vi "Initialize Instrument.vi"(8 "error in (no error)":errorcluster, 10 "Reset":bool, 11 "RS Z2X in":refnum<class "RS Z2X.lvclass">) -> (0 "error out":errorcluster, 3 "RS Z2X out":refnum<class "RS Z2X.lvclass">)   [LabVIEW 2020, in "RS Z2X.lvclass"]
uses:
  RS Z2X.lvclass
  C:/Sandbox/RF Bench/Source Code/WiSpry Test Framework/Instruments/Instrument.lvclass
  Instrument.lvclass/Instrument.ctl
  <vilib>/Instr/_visa.llb/VISA Open Access Mode.ctl
  Instrument.lvclass
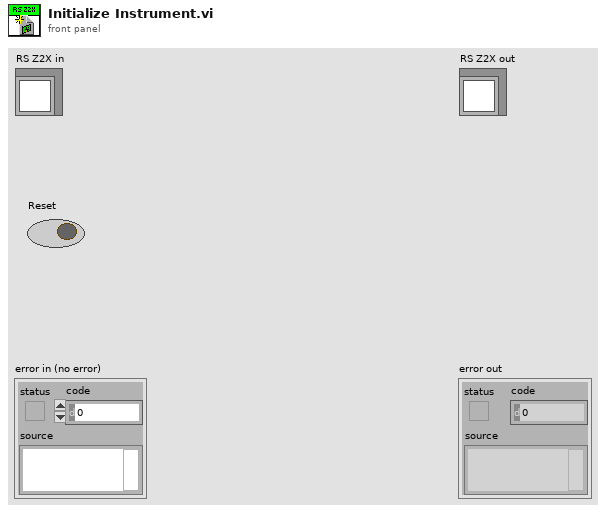
[diagram p1: front panel]
types:
  T1 = typedef "VISA Open Access Mode.ctl" = u32
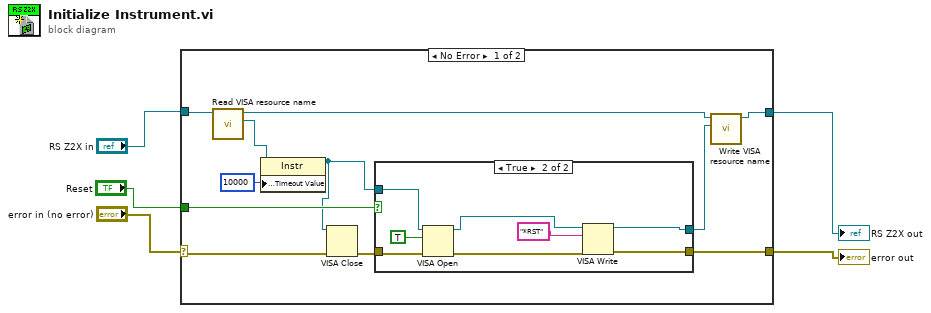
[diagram p0: block diagram]
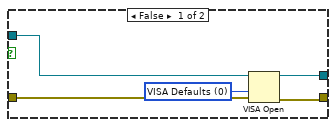
[diagram p2: hidden frame]
diagram:
  n1 = case shown="No Error" "error in (no error)" {
    selector: "error in (no error)" -> [w6 w31]
    tunnel: [w15 w31] -> w2
    tunnel: "RS Z2X in" -> [w16 w30]
    tunnel: [w10 w30] -> w1
    tunnel: "Reset" -> [w14 _]
    frame No Error {
      n2 = call "Read VISA resource name.vi"("Instrument in"=w16) -> ("VISA resource name"=w12:refnum<visa-resource-name>, "Instrument out"=w11:refnum<class "RS Z2X.lvclass">)  [unwired: 9 in]
      n3 = property class="Instr"(reference=w12, "General Settings:Timeout Value"=u32 10000) -> (reference out=w7:refnum<visa-resource-name>)  [unwired: 1 in, 1 out]
      n4 = VISA Close(VISA resource name=w7, error in (no error)=w6) -> (error out=w8:errorcluster)
      n5 = case shown="True" w14 {
        tunnel: [w21 w23] -> w15
        tunnel: w7 -> [w19 w27]
        tunnel: w8 -> [w18 w28]
        tunnel: [w20 w22] -> w9
        frame False {
          w17 = T1 0 items=["VISA Defaults"=0, "Exclusive Lock"=1, "Load Configured Settings"=4] ("Access Mode")
          n6 = VISA Open(access mode=w17, error in (no error)=w18, VISA resource name=w19) -> (VISA resource name=w20:refnum<visa-resource-name>, error out=w21:errorcluster)  [unwired: 2 in]
        }
        frame True {
          n7 = VISA Open(duplicate session (F)=TRUE, error in (no error)=w28, VISA resource name=w27) -> (VISA resource name=w25:refnum<visa-resource-name>, error out=w26:errorcluster)  [unwired: 2 in]
          n8 = VISA Write(VISA resource name=w25, write buffer="*RST", error in (no error)=w26) -> (VISA resource name out=w22:refnum<visa-resource-name>, error out=w23:errorcluster)  [unwired: 1 out]
        }
      }
      n9 = call "Write VISA resource name.vi"("VISA resource name"=w9, "Instrument in"=w11) -> ("Instrument out"=w10:refnum<class "RS Z2X.lvclass">)  [unwired: 9 in]
    }
    frame Error {
    }
  }
  "error out" <- w2
  "RS Z2X out" <- w1
